vi "Stop Core.vi"(10 "final error code":i32, 11 "Display Panel V3 in":refnum<class "Display Panel V3.lvclass">) -> (3 "Display Panel V3 out":refnum<class "Display Panel V3.lvclass">)   [LabVIEW 2013]
doc: "(<B>Filename</B>: Actor Framework.lvlib:Actor.lvclass:Stop Core.vi)\n\nDefines what the actor does before it stops. Use the <B>final error code</B> input to determine whether the actor shut down in response to an error.\n\nBy default, this method does nothing. A descendant class may override it to define behavior, such as shutting down any processes the actor initiated in its override of the Actor Core method."
uses:
  Display Panel V3.lvclass
panel:
  out "error out":errorcluster
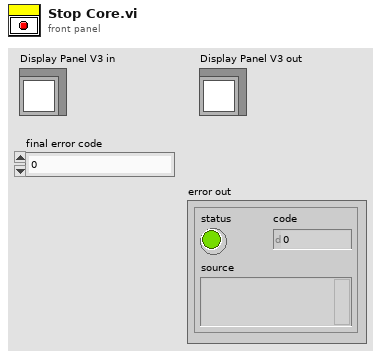
[diagram p1: front panel]
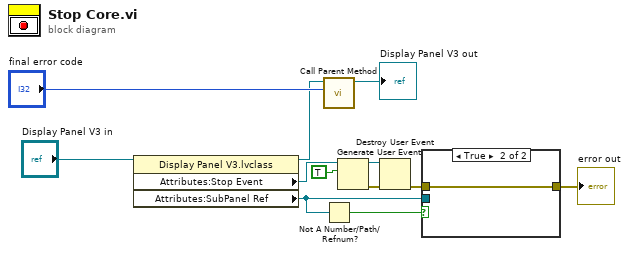
[diagram p0: block diagram]
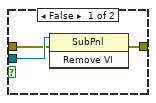
[diagram p2: hidden frame]
diagram:
  n1 = property class="Display Panel V3.lvclass"(reference="Display Panel V3 in") -> (reference out=w3:refnum<class "Display Panel V3.lvclass">, "Attributes:Stop Event"=w7:refnum<user-event>, "Attributes:SubPanel Ref"=w5:refnum<vi>)  [unwired: 1 in, 1 out]
  n2 = call-parent "Call Parent Method"("final error code"="final error code", "Actor in"=w3) -> ("Actor out"=→"Display Panel V3 out":refnum<class "Display Panel V3.lvclass">)  [unwired: 9 in]
  n3 = Not A Number/Path/Refnum?(number/path/refnum=w5) -> (NaN/Path/Refnum?=w6:bool)
  n4 = Generate User Event(user event=w7, event data cluster=TRUE ("event data")) -> (user event out=w9:refnum<user-event>, error out=w10:errorcluster)  [unwired: 2 in]
  n5 = Destroy User Event(user event=w9, error in=w10) -> (error out=w4:errorcluster)
  n6 = case shown="True" w6 {
    tunnel: w5 -> [w15 _]
    tunnel: w4 -> [w14 w16]
    tunnel: [w13 w16] -> w1
    frame False {
      n7 = invoke class="SubPnl" method="Remove VI"(reference=w15, error in=w14) -> (error out=w13:errorcluster)  [unwired: 1 in, 2 out]
    }
    frame True {
    }
  }
  "error out" <- w1
